vi "upload.tdms.vi"(8 "error in":errorcluster, 9 "timeout per chunk (ms)":i32=300000, 10 "File Path":path, 11 "Nominal Client in":refnum<class "Nominal Client.lvclass">) -> (0 "error out":errorcluster, 3 "Nominal Client out":refnum<class "Nominal Client.lvclass">)   [LabVIEW 2020, in "Nominal Client.lvclass"]
doc: "This VI uploads a specified TDMS file to the Nominal platform. Only channels containing waveform data types are uploaded, ensuring that other unsupported data types are ignored. All properties associated with the waveform channels are preserved and uploaded alongside the data. The VI waits for the Nominal platform to fully ingest the TDMS file before completing its execution, ensuring data integrity and confirmation of successful upload."
uses:
  Nominal Client.lvclass
  Nominal Client.lvclass/Nominal Client.ctl
  catalog.wait_until_multiple_ingest_complete.vi
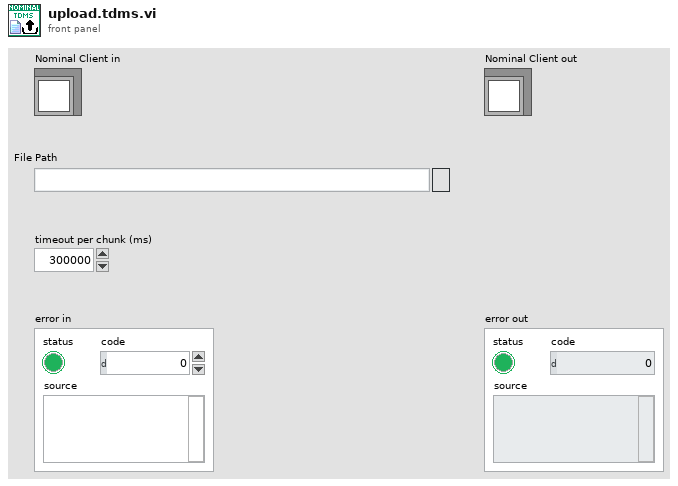
[diagram p1: front panel]
types:
  T1 = enum16{"open", "open or create", "create or replace", "create", "open (read-only)"}
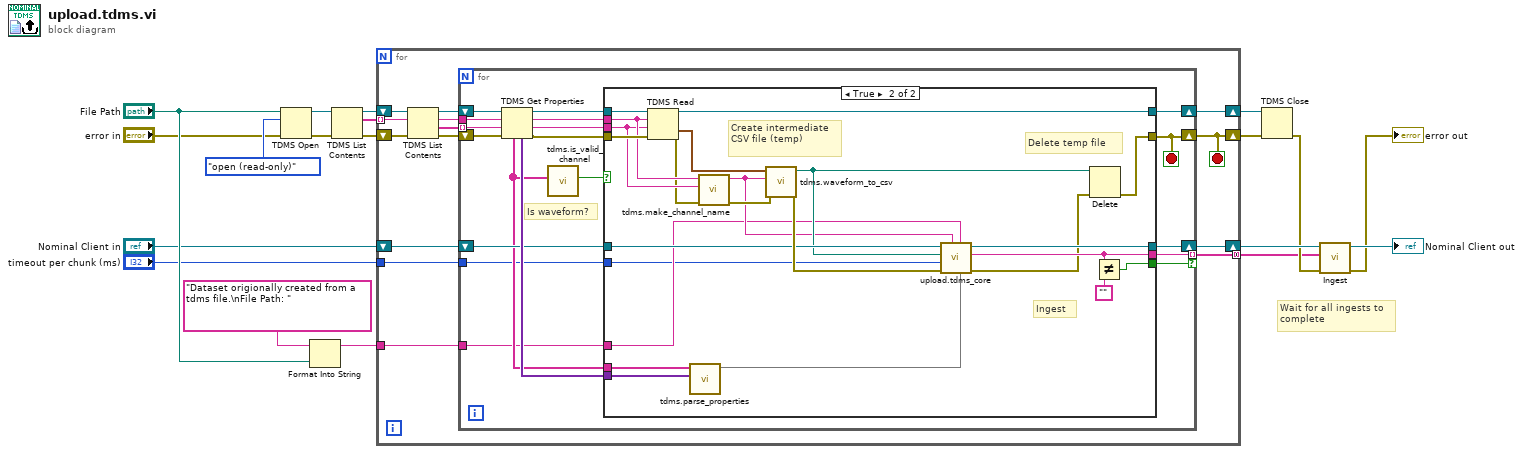
[diagram p0: block diagram]
diagram:
  # "Wait for all ingests to complete"
  n1 = TDMS Open(8:"error in", 10:T1."open (read-only)" ("operation (0:open)"), 11:"File Path") -> (0:w18:errorcluster, 3:w19:refnum<k34>)  [unwired: 4 in]
  n2 = Format Into String(initial string="Dataset origionally created from a tdms file.\nFile Path: ", "File Path") -> (resulting string=w8:string)  [unwired: 2 in, 1 out]
  n3 = TDMS List Contents(4:w18, 7:w19) -> (0:w5:errorcluster, 2:w14:string[], 3:w17:refnum<k34>)  [unwired: 1 in, 1 out]
  n4 = for {
    shift-right: [w26] -> w15
    shift-left: w17 -> [w33]
    shift-right: [w21] -> w16
    shift-left: w5 -> [w32]
    tunnel: w14 -> [w31] mode=indexing
    shift-right: [w25] -> w13
    shift-left: "Nominal Client in" -> [w24]
    tunnel: [w23] -> w7 mode=concatenating
    tunnel: w8 -> [w22]
    tunnel: "timeout per chunk (ms)" -> [w20]
    stop <- w21 stop-if-true
    n5 = TDMS List Contents(4:w32, 6:w31, 7:w33) -> (0:w27:errorcluster, 1:w28:string[], 2:w29:string, 3:w30:refnum<k34>)
    n6 = for {
      tunnel: w29 -> [w49]
      tunnel: w28 -> [w48] mode=indexing
      shift-right: [w35] -> w21
      shift-left: w27 -> [w51]
      shift-right: [w45] -> w26
      shift-left: w30 -> [w52]
      shift-right: [w42] -> w25
      shift-left: w24 -> [w41]
      tunnel: [w38] -> w23 mode=indexing if=w37
      tunnel: w22 -> [w36]
      tunnel: w20 -> [w34]
      stop <- w35 stop-if-true
      # "Is waveform?"
      n7 = TDMS Get Properties(8:w51, 9:w48, 10:w49, 11:w52) -> (0:w46:errorcluster, 1:w43:string, 2:w44:string, 3:w47:refnum<k34>, 4:w50:variant[], 6:w40:string[])  [unwired: 2 in]
      n8 = call "tdms.is_valid_channel.vi"("TDMS Property Names"=w40) -> ("Valid Channel"=w39:bool)  [unwired: 10 in]
      n9 = case shown="True" w39 {
        tunnel: w50 -> [_ w71]
        tunnel: w40 -> [_ w72]
        tunnel: w47 -> [w55 w78]
        tunnel: w46 -> [w54 w77]
        tunnel: [w55 w76] -> w45
        tunnel: [w54 w66] -> w35
        tunnel: w44 -> [_ w74]
        tunnel: w43 -> [_ w73]
        tunnel: [w53 w64] -> w42
        tunnel: w41 -> [w53 w61]
        tunnel: [_ w65] -> w38
        tunnel: [_ w69] -> w37
        tunnel: w36 -> [_ w58]
        tunnel: w34 -> [_ w56]
        frame False {
        }
        frame True {
          # "Ingest"
          # "Delete temp file"
          # "Create intermediate CSV file (temp)"
          n10 = TDMS Read(0:w78, 5:w74, 7:w73, 11:w77) -> (4:w76:refnum<k34>, 10:w75:waveform(dbl), 15:w67:errorcluster)  [unwired: 4 in, 3 out]
          n11 = call "tdms.parse_properties.vi"("Property Values"=w71, "Property Names"=w72) -> ("Property Map"=w57:map{string, string})  [unwired: 9 in]
          n12 = call "tdms.make_channel_name.vi"("error in"=w67, "Channel Name"=w73, "Group Name"=w74) -> ("error out"=w70:errorcluster, "channel name"=w59:string)  [unwired: 7 in]
          n13 = call "tdms.waveform_to_csv.vi"("error in"=w70, "Formatted Channel Name"=w59, "Waveform"=w75) -> ("error out"=w62:errorcluster, "new csv filepath"=w60:path)  [unwired: 7 in]
          n14 = call "upload.tdms_core.vi"("Properties"=w57, "Description"=w58, "Name"=w59, "error in"=w62, "timeout (ms)"=w56, "File Path"=w60, "Nominal Client in"=w61) -> ("error out"=w63:errorcluster, "datasetRID"=w65:string, "Nominal Client out"=w64:refnum<class "Nominal Client.lvclass">)  [unwired: 2 in]
          n15 = Delete(path (use dialog)=w60, error in=w63) -> (error out=w66:errorcluster)  [unwired: 3 in, 2 out]
          n16 = Not Equal?(x=w65, y="") -> (x != y?=w69:bool)
        }
      }
    }
  }
  n17 = TDMS Close(8:w16, 11:w15) -> (0:w12:errorcluster)  [unwired: 1 out]
  n18 = call-poly "Ingest.vi"("error in"=w12, "datasetRid"=w7, "Nominal Client"=w13) -> ("error out"=→"error out":errorcluster, "Nominal Client out"=→"Nominal Client out":refnum<class "Nominal Client.lvclass">)  [unwired: 7 in]
